vi "read_CurrentLimit_subvi.vi"(8 "error in (no error)":errorcluster, 10 "Address (0x50)":u16=80 max=1023 format="%.0x", 11 "Aardvark Handle":i32 min=0) -> (0 "error out":errorcluster, 2 "Current":dbl, 3 "Dup Aardvark Handle":i32)   [LabVIEW 2014]
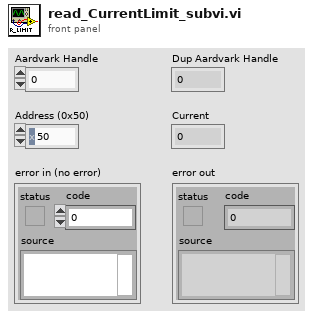
[diagram p1: front panel]
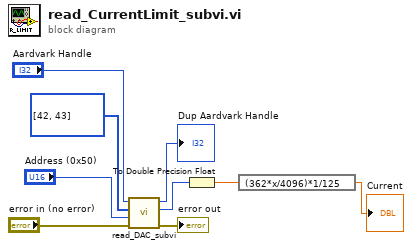
[diagram p0: block diagram]
diagram:
  n1 = call "read_DAC_subvi.vi"("error in (no error)"="error in (no error)", "Address (0x50)"="Address (0x50)", "DAC_ADD"=u8[] [42, 43], "Aardvark Handle"="Aardvark Handle") -> ("error out"=→"error out":errorcluster, "DAC Val"=w8:u16, "Dup Aardvark Handle"=→"Dup Aardvark Handle":i32)  [unwired: 3 in]
  n2 = To Double Precision Float(number=w8) -> (double precision float=w1:dbl)
  n3 = expression code="(362*x/4096)*1/125"(w1) -> (→"Current":dbl)
